vi "labview串口-5.vi"() -> ()   [LabVIEW 2018]
uses:
  <vilib>/Instr/_visa.llb/VISA Configure Serial Port (Instr).vi
panel:
  in  "发送":bool
  out "读取缓冲区 2":string
  out "读取字节数2":u32
  in  "读取":bool
  in  "等待时间":u32
  in  "flow control (0:none) 2":u16(ring) caption="流程控制" items=["无", "XON/XOFF", "RTS/CTS", "XON/XOFF & RTS/CTS", "DTR/DSR", "XON/XOFF & DTR/DSR"]
  in  "stop bits (10: 1 bit) 2":u16(ring)=10 caption="停止位" items=["1.0"=10, "1.5"=15, "2.0"=20]
  in  "parity (0:none) 2":enum16{"None", "Odd", "Even", "Mark", "Space"}(ring) caption="奇偶"
  in  "data bits (8) 2":u16=8 caption="数据比特" min=5 max=8 step=1
  in  "baud rate (9600) 2":u32=9600 caption="波特率"
  in  "VISA resource name 2":refnum<visa-resource-name> caption="VISA资源名称"
  in  "timeout (10sec) 2":u32=10000 caption="超时（10秒）"
  in  "启用终止符 2":bool=TRUE caption="启用终止\n符 (T)"
  in  "雷达俯仰":bool
  in  "测量按钮":bool
  in  "雷达偏航":u8(slide) scale=1.0..20.0
  in  "油门":u16(slide) scale=0.0..10.0
  in  "进退":u16(slide) scale=0.0..10.0
  in  "偏航":u16(slide) scale=0.0..10.0
  in  "平移":u16(slide) scale=0.0..10.0
  in  "自动（雷达）":bool
  in  "360°翻转":bool
  out "读取的字节":u32
  out "读取缓冲区":string
  in  "读取前延时（ms)":u32
  in  "flow control (0:none)":u16(ring) caption="流程控制" items=["无", "XON/XOFF", "RTS/CTS", "XON/XOFF & RTS/CTS", "DTR/DSR", "XON/XOFF & DTR/DSR"]
  in  "stop bits (10: 1 bit)":u16(ring)=10 caption="停止位" items=["1.0"=10, "1.5"=15, "2.0"=20]
  in  "parity (0:none)":enum16{"None", "Odd", "Even", "Mark", "Space"}(ring) caption="奇偶"
  in  "data bits (8)":u16=8 caption="数据比特" min=5 max=8 step=1
  in  "baud rate (9600)":u32=9600 caption="波特率"
  in  "VISA resource name":refnum<visa-resource-name> caption="VISA资源名称"
  in  "读取":bool
  in  "写入":bool
  in  "写入字符串":string
  in  "timeout (10sec)":u32=10000 caption="超时（10秒）"
  in  "启用终止符":bool=TRUE caption="启用终止\n符 (T)"
  # "雷达控制指令自动发射及雷达探测信息接收窗口"
  # "无人机/雷达控制器"
  # "无人机飞行指令发送窗口"
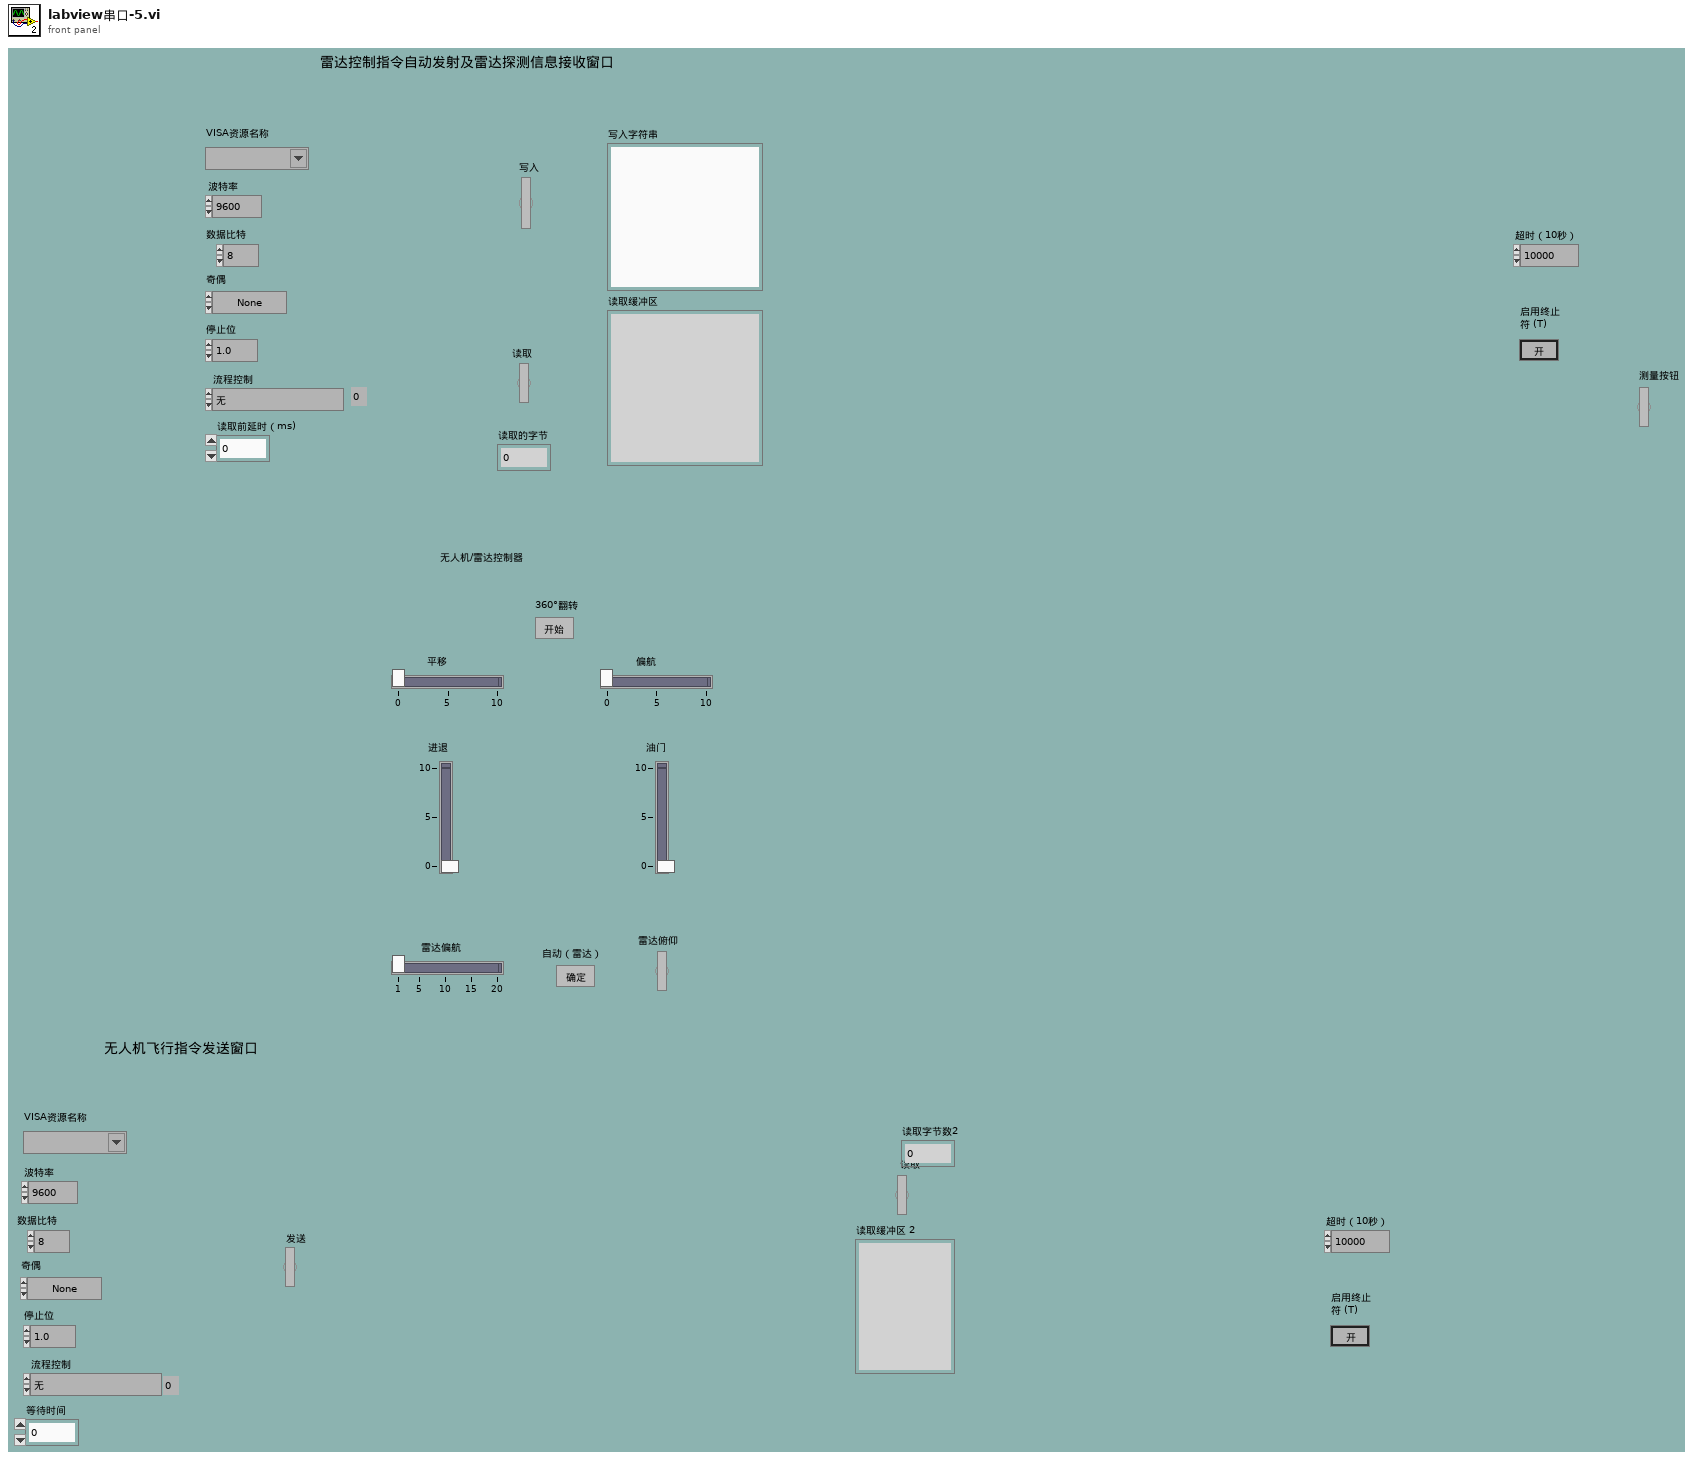
[diagram p1: front panel]
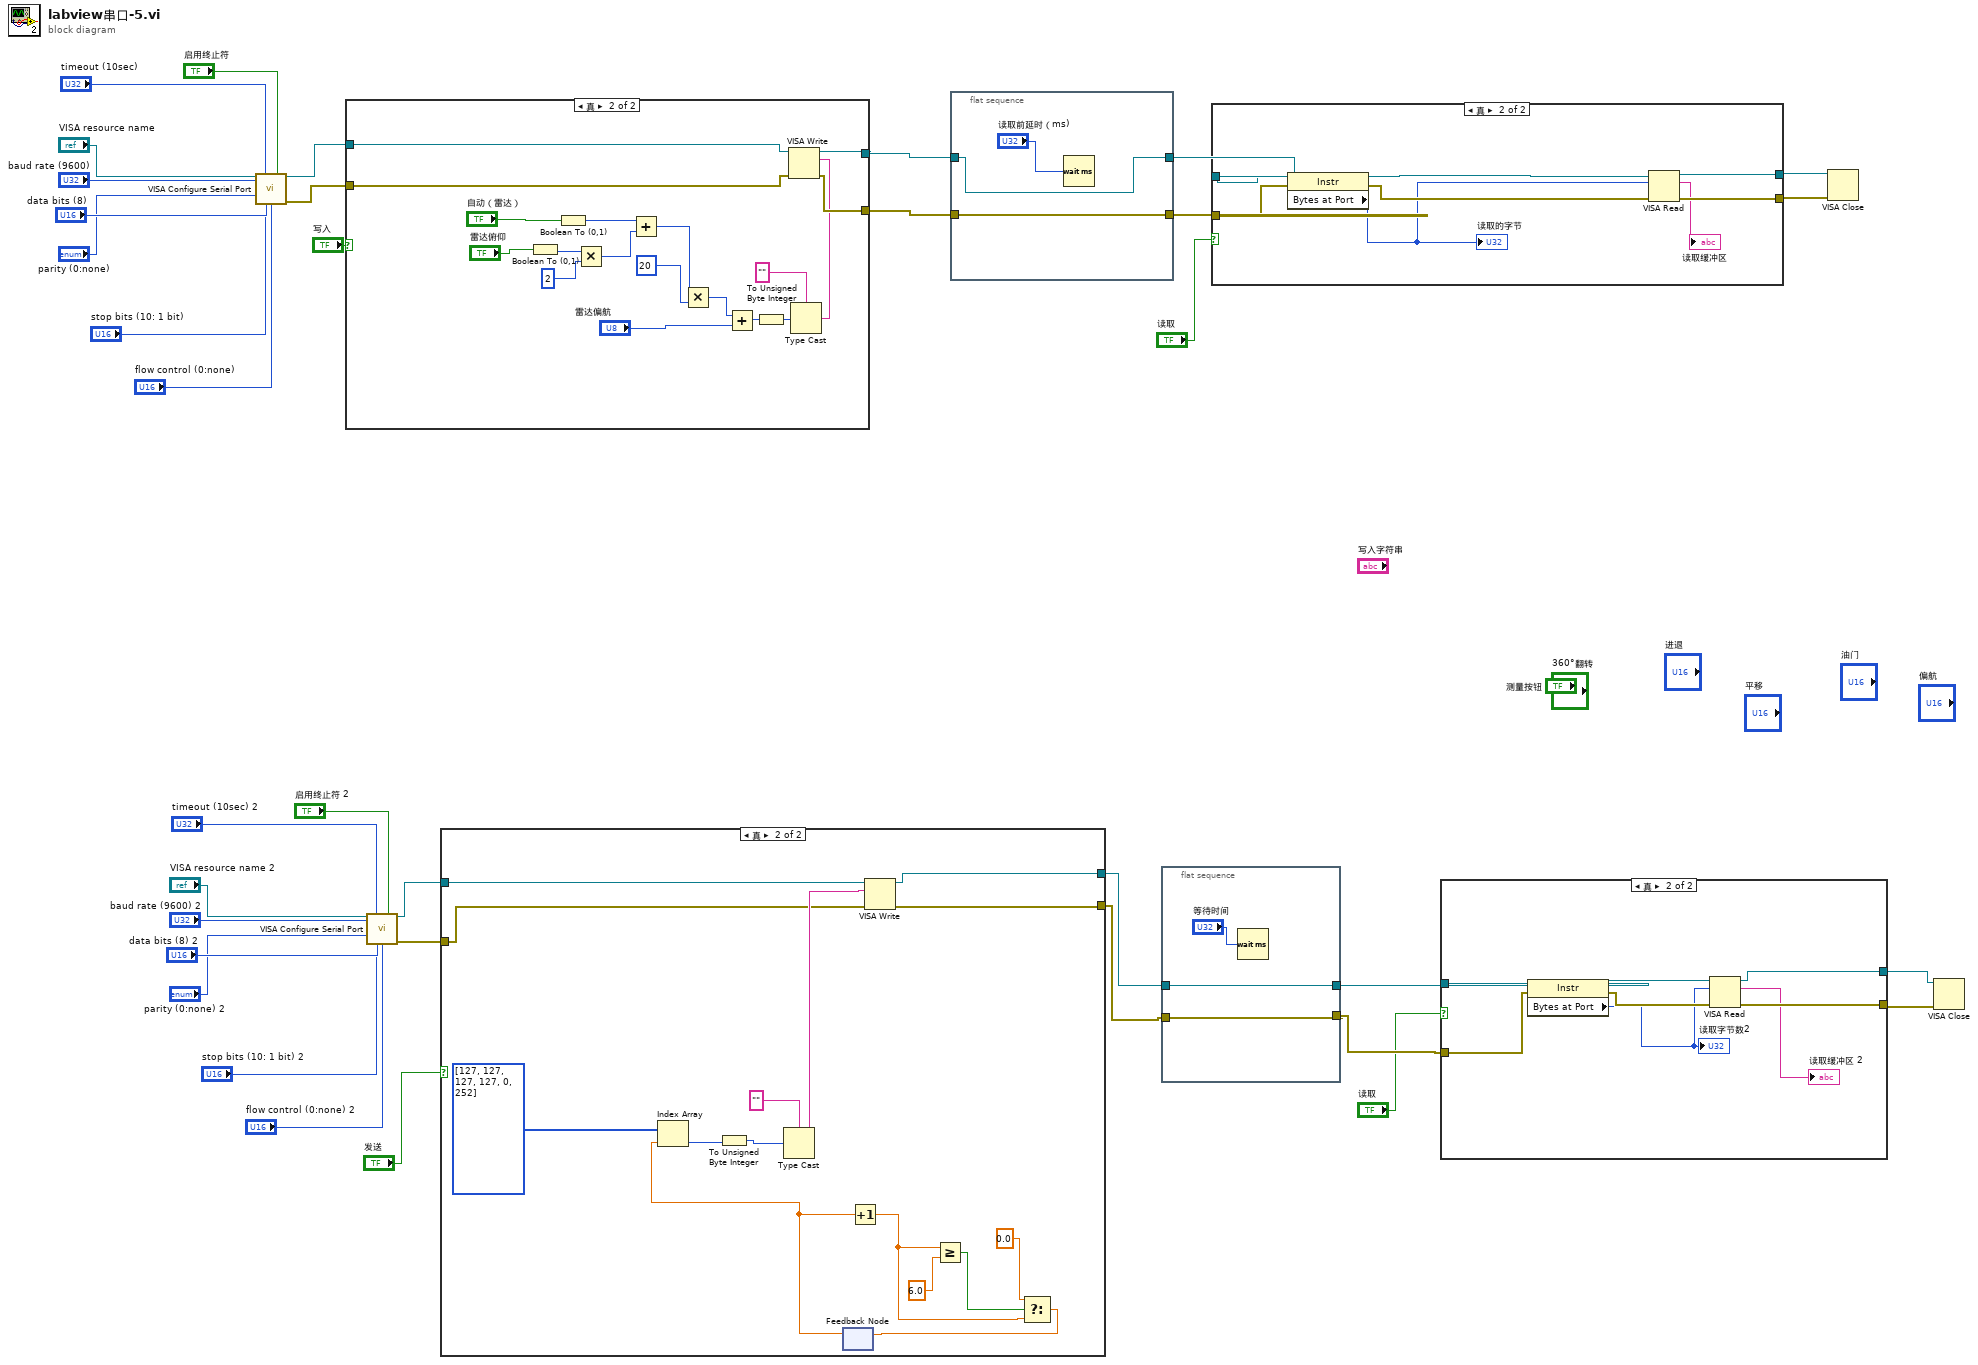
[diagram p0: block diagram]
diagram:
  n1 = call-poly "VISA Configure Serial Port"("VISA resource name"="VISA resource name", "timeout (10sec)"="timeout (10sec)", "Enable Termination\nChar (T)"="启用终止符", "baud rate (9600)"="baud rate (9600)", "data bits (8)"="data bits (8)", "parity (0:none)"="parity (0:none)", "stop bits (10: 1 bit)"="stop bits (10: 1 bit)", "flow control (0:none)"="flow control (0:none)") -> ("VISA resource name out"=w34:refnum<visa-resource-name>, "error out"=w33:errorcluster)  [unwired: 6 in]
  n2 = case shown="真" "写入" {
    tunnel: w34 -> [w38 w56]
    tunnel: w33 -> [w37 w55]
    tunnel: [w38 w54] -> w32
    tunnel: [w37 w53] -> w31
    frame False {
    }
    frame True {
      n3 = Boolean To (0,1)(Boolean="雷达俯仰") -> (0, 1=w48:i16)
      n4 = Boolean To (0,1)(Boolean="自动（雷达）") -> (0, 1=w49:i16)
      n5 = Multiply(x=w48, y=2) -> (x*y=w46:i32)
      n6 = Add(x=w49, y=w46) -> (x+y=w50:i32)
      n7 = Multiply(x=w50, y=u8 20) -> (x*y=w44:i32)
      n8 = Add(x=w44, y="雷达偏航") -> (x+y=w39:i32)
      n9 = To Unsigned Byte Integer(number=w39) -> (unsigned 8bit integer=w40:u8)
      n10 = Type Cast(type="", x=w40) -> (*(type *) &x=w41:string)
      n11 = VISA Write(VISA resource name=w56, write buffer=w41, error in (no error)=w55) -> (VISA resource name out=w54:refnum<visa-resource-name>, error out=w53:errorcluster)  [unwired: 1 out]
    }
  }
  n12 = call-poly "VISA Configure Serial Port"("VISA resource name"="VISA resource name 2", "timeout (10sec)"="timeout (10sec) 2", "Enable Termination\nChar (T)"="启用终止符 2", "baud rate (9600)"="baud rate (9600) 2", "data bits (8)"="data bits (8) 2", "parity (0:none)"="parity (0:none) 2", "stop bits (10: 1 bit)"="stop bits (10: 1 bit) 2", "flow control (0:none)"="flow control (0:none) 2") -> ("VISA resource name out"=w8:refnum<visa-resource-name>, "error out"=w9:errorcluster)  [unwired: 6 in]
  n13 = case shown="真" "发送" {
    tunnel: w8 -> [_ w58]
    tunnel: [_ w71] -> w7
    tunnel: [_ w70] -> w6
    tunnel: w9 -> [_ w59]
    frame False {
    }
    frame True {
      n14 = feedback #1() -> (w64:dbl)  [unwired: 1 in]
      n15 = Index Array(array=i32[] [127, 127, 127, 127, 0, 252], index=w64) -> (element=w63:i32)
      n16 = To Unsigned Byte Integer(number=w63) -> (unsigned 8bit integer=w62:u8)
      n17 = Type Cast(type="", x=w62) -> (*(type *) &x=w60:string)
      n18 = Increment(x=w64) -> (x+1=w66:dbl)
      n19 = VISA Write(VISA resource name=w58, write buffer=w60, error in (no error)=w59) -> (VISA resource name out=w71:refnum<visa-resource-name>, error out=w70:errorcluster)  [unwired: 1 out]
      n20 = Greater Or Equal?(x=w66, y=6.0) -> (x >= y?=w65:bool)
      n21 = Select(t=0.0, s=w65, f=w66) -> (s? t:f=w57:dbl)
      n22 = feedback-in #1(w57) -> ()
    }
  }
  n23 = flat-sequence {
    tunnel: w32 -> [w74]
    tunnel: w31 -> [w73]
    tunnel: [w74] -> w30
    tunnel: [w73] -> w29
    frame #0 {
      n24 = Wait (ms)(milliseconds to wait="读取前延时（ms)") -> ()  [unwired: 1 out]
    }
  }
  n25 = flat-sequence {
    tunnel: w7 -> [w75]
    tunnel: w6 -> [w76]
    tunnel: [w75] -> w10
    tunnel: [w76] -> w5
    frame #0 {
      n26 = Wait (ms)(milliseconds to wait="等待时间") -> ()  [unwired: 1 out]
    }
  }
  n27 = case shown="真" "读取" {
    tunnel: w30 -> [w79 w87]
    tunnel: w29 -> [w78 w86]
    tunnel: [w79 w83] -> w13
    tunnel: [w78 w82] -> w12
    frame False {
    }
    frame True {
      n28 = property class="Instr"(reference=w87, error in=w86) -> (reference out=w84:refnum<visa-resource-name>, error out=w85:errorcluster, "Bytes at Port"=w80:u32)
      "读取的字节" <- w80
      n29 = VISA Read(VISA resource name=w84, byte count=w80, error in (no error)=w85) -> (VISA resource name out=w83:refnum<visa-resource-name>, read buffer=→"读取缓冲区":string, error out=w82:errorcluster)  [unwired: 1 out]
    }
  }
  n30 = case shown="真" "读取" {
    tunnel: w5 -> [_ w95]
    tunnel: w10 -> [_ w94]
    tunnel: [_ w93] -> w3
    tunnel: [_ w89] -> w2
    frame False {
    }
    frame True {
      n31 = property class="Instr"(reference=w94, error in=w95) -> (reference out=w92:refnum<visa-resource-name>, error out=w91:errorcluster, "Bytes at Port"=w90:u32)
      "读取字节数2" <- w90
      n32 = VISA Read(VISA resource name=w92, byte count=w90, error in (no error)=w91) -> (VISA resource name out=w93:refnum<visa-resource-name>, read buffer=→"读取缓冲区 2":string, error out=w89:errorcluster)  [unwired: 1 out]
    }
  }
  n33 = VISA Close(VISA resource name=w13, error in (no error)=w12) -> ()  [unwired: 1 out]
  n34 = VISA Close(VISA resource name=w3, error in (no error)=w2) -> ()  [unwired: 1 out]
